vi "funçãoAvaliaçãoAtacante.vi"(9 "balls":T9[](array[typedef]), 10 "Robot in":T4, 11 "IA State":T3={"our_robots"=[], "enemy_robots"=[], "balls"=[], "geometry"={"field_length"=0, "field_width"=0, "goal_width"=0, "goal_depth"=0, "center_circle_radius"=0, "defense_width"=0, "defense_depth"=0, "free_kick_from_defense_dist"=0, "penalty_spot_from_field_line_dist"=0, "penalty_line_from_spot_dist"=0, "half_moon_depth"=0, "half_moon_width"=0}, "IA Judge"={"stage"="", "command"="", "our_goalie_id"=0.0, "enemy_goalie_id"=0.0, "command enum"=enum."Halt", "Time"=enum."Azul"}, "Received Timestamp"=timestamp(0 s since 1904-01-01), "Events"={"Touch"=FALSE, "id touch"=0.0, "Ball out of \nVision"=FALSE, "Ball inside \nGoalie area"=FALSE, "Robot not responding"=FALSE, "Robots responding status"=[1.0, 1.0, 1.0, 1.0, 1.0, 1.0], "Enemy Ball \nPossession"=FALSE, "Id ini Possession"=0.0, "Ball Possesion"=FALSE, "Id Possesion"=0.0, "Ball at\nour goal side"=FALSE, "Ball at\ntouchline"=FALSE, "Ball at\nenemy goal side"=FALSE}}) -> (2 "Parede":T1(ring), 3 "Estado_Atacante":T2(ring))   [LabVIEW 2018]
doc: "Função que avalia o estado do atacante,"
uses:
  Intel/Functions Enum.ctl
  Intel/AttackerStates.ctl
  Path Planning/RRT/PathDest.ctl
  Path Planning/RRT/PathDests.ctl
  Core/AI Robot.ctl
  Core/AI Ball.ctl
  Core/Field Size.ctl
  Intel/Command Enum.ctl
  Core/AI Judge.ctl
  Util/Events/Events.ctl
  Core/AI Input.ctl
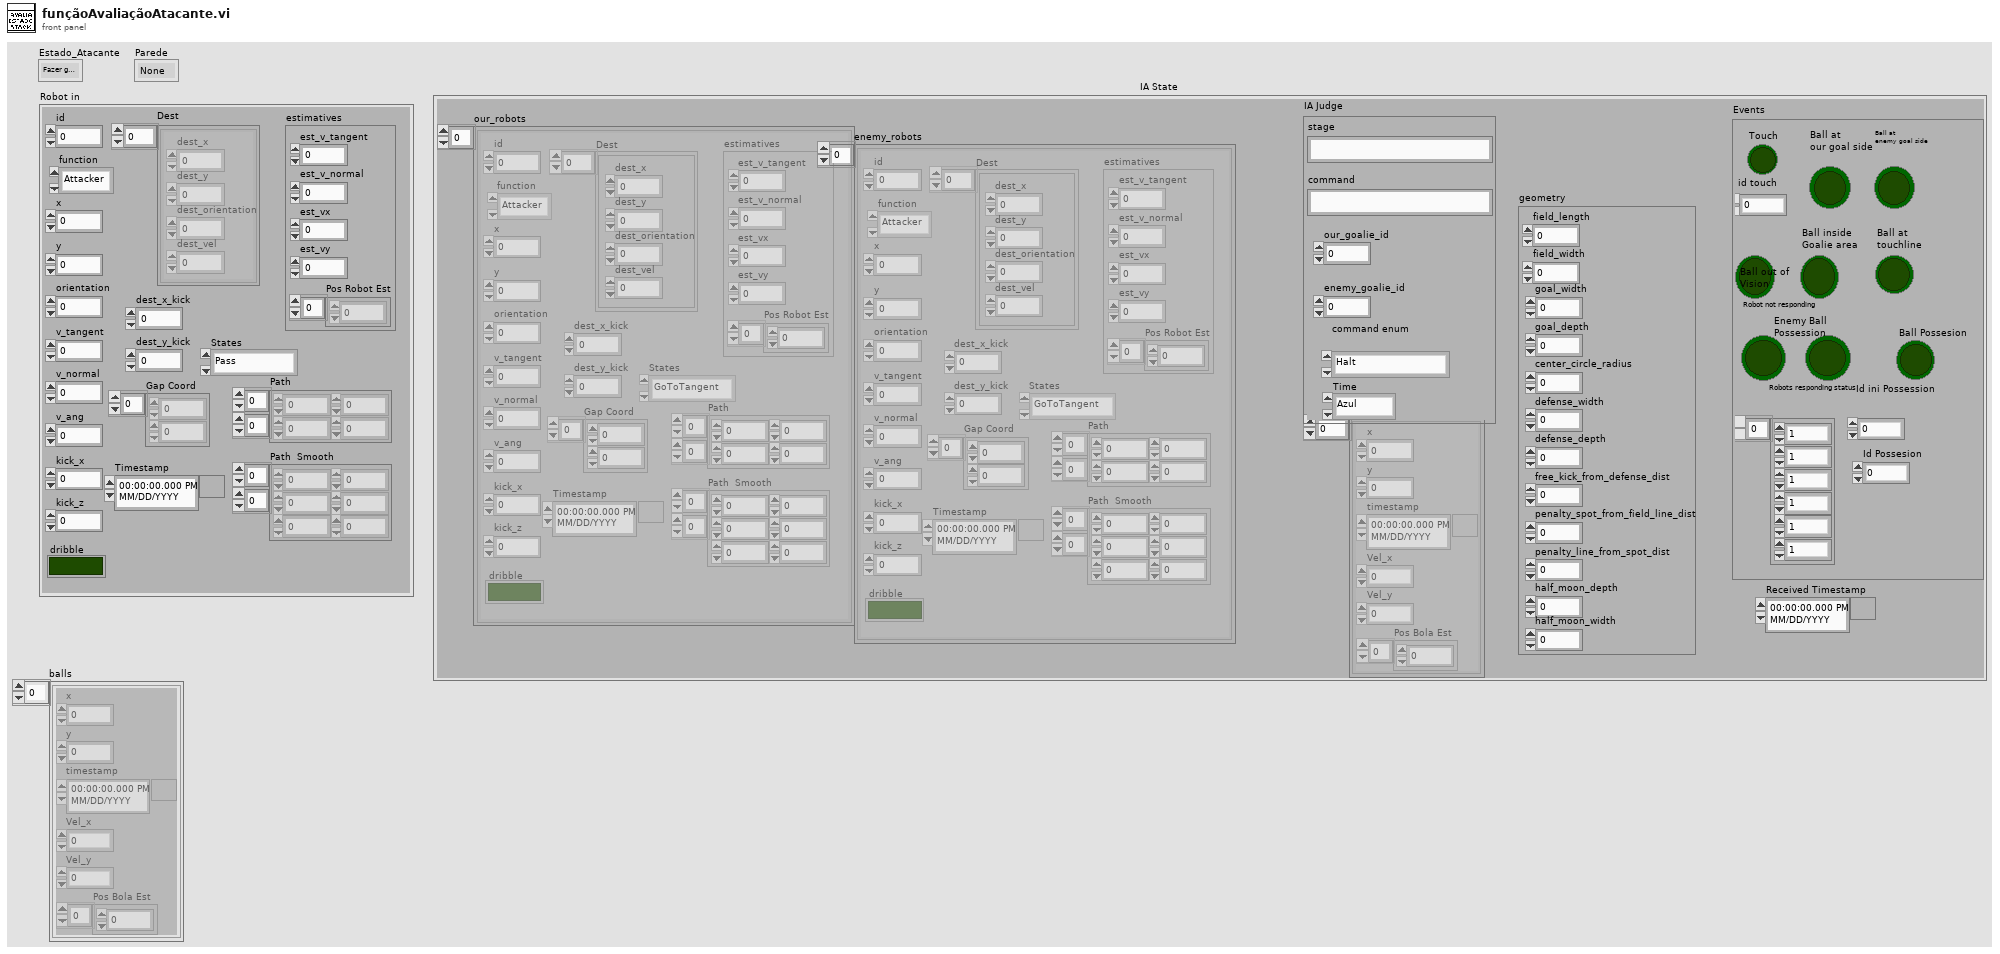
[diagram p1: front panel]
types:
  T1 = enum16{"None", "Frente", "Trás", "Cima", "Baixo"}
  T2 = enum16{"Fazer gol pela lateral", "Tirar bola da parede", "Default", "Sair da parede", "Spin igual a um louco"}
  T3 = typedef "AI Input.ctl" = cluster{"our_robots":T4[], "enemy_robots":T4[], "balls":T9[], "geometry":T10, "IA Judge":T11, "Received Timestamp":timestamp, "Events":T13}
  T4 = typedef "AI Robot.ctl" = cluster{"id":u32, "function":T5, "x":dbl, "y":dbl, "orientation":dbl, "v_tangent":dbl, "v_normal":dbl, "v_ang":dbl, "kick_x":dbl, "kick_z":dbl, "dribble":bool, "Timestamp":timestamp, "estimatives":cluster{"est_v_tangent":dbl, "est_v_normal":dbl, "est_vx":dbl, "est_vy":dbl, "Pos Robot Est":dbl[]}, "dest_x_kick":dbl, "dest_y_kick":dbl, "Gap Coord":dbl[], "States":T6, "Path ":dbl[][], "Path  Smooth":dbl[][], "Dest":T7}
  T5 = typedef "Functions Enum.ctl" = enum16{"Attacker", "Goalie", "Defender", "Striker", "Goto 0", "Dummy", "Kicker", "ZigZag"}
  T6 = typedef "AttackerStates.ctl" = enum16{"Pass", "GoToTangent", "BallGetting", "GoToKick", "Rotate anti-clockwise", "Rotate Clockwise", ""}
  T7 = typedef "PathDests.ctl" = T8[]
  T8 = typedef "PathDest.ctl" = cluster{"dest_x":dbl, "dest_y":dbl, "dest_orientation":dbl, "dest_vel":dbl}
  T9 = typedef "AI Ball.ctl" = cluster{"x":dbl, "y":dbl, "timestamp":timestamp, "Vel_x":dbl, "Vel_y":dbl, "Pos Bola Est":dbl[]}
  T10 = typedef "Field Size.ctl" = cluster{"field_length":u32, "field_width":u32, "goal_width":u32, "goal_depth":u32, "center_circle_radius":u32, "defense_width":u32, "defense_depth":u32, "free_kick_from_defense_dist":u32, "penalty_spot_from_field_line_dist":u32, "penalty_line_from_spot_dist":u32, "half_moon_depth":u32, "half_moon_width":u32}
  T11 = typedef "AI Judge.ctl" = cluster{"stage":string, "command":string, "our_goalie_id":dbl, "enemy_goalie_id":dbl, "command enum":T12, "Time":enum16{"Azul", "Amarelo"}}
  T12 = typedef "Command Enum.ctl" = enum16{"Halt", "Stop", "Force Start", "PKA Normal Start", "Prepare Kickoff Ally", "PKE Normal Start", "Prepare Kickoff Enemy", "Prepare Penalty Ally", "PPA Normal Start", "Prepare Penalty Enemy", "PPE Normal Start", "Ball Placement Enemy Up", "Ball Placement Enemy Down", "Ball Placement Ally Up", "Ball Placement Ally Mid", "Ball Placement Ally Down", "Indirect Free Enemy", "Indirect Free Ally", "Timeout Enemy", "Timeout Ally", "Goal Enemy", "Goal Ally", "Normal Half Time", "Extra Time Break", "Extra Half Time", "None", "Post Game"}
  T13 = typedef "Events.ctl" = cluster{"Touch":bool, "id touch":dbl, "Ball out of \nVision":bool, "Ball inside \nGoalie area":bool, "Robot not responding":bool, "Robots responding status":dbl[], "Enemy Ball \nPossession":bool, "Id ini Possession":dbl, "Ball Possesion":bool, "Id Possesion":dbl, "Ball at\nour goal side":bool, "Ball at\ntouchline":bool, "Ball at\nenemy goal side":bool}
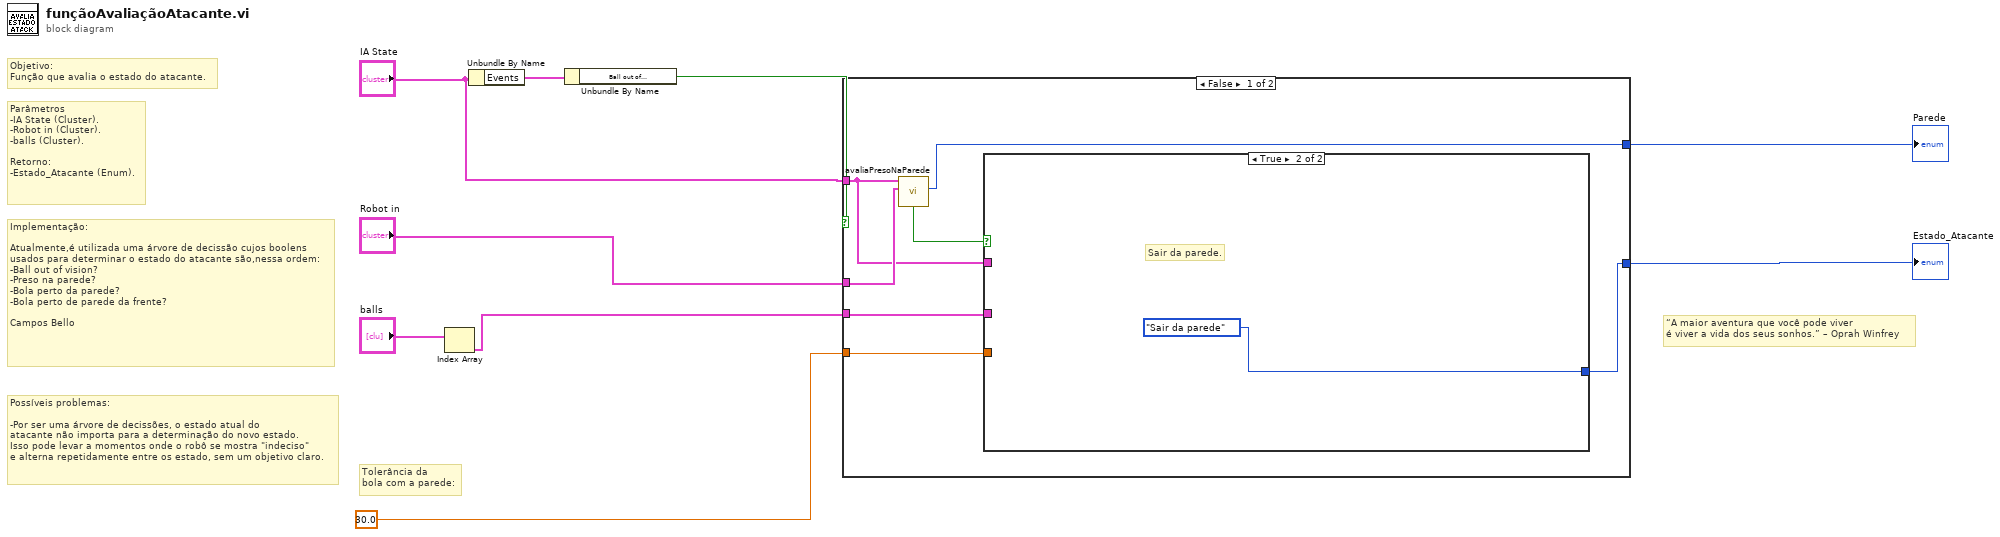
[diagram p0: block diagram]
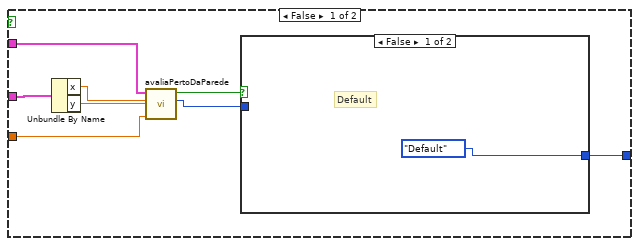
[diagram p2: hidden frame]
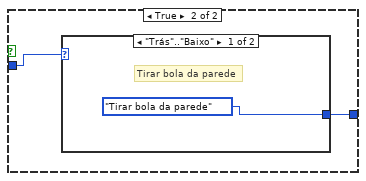
[diagram p3: hidden frame]
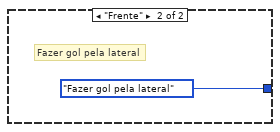
[diagram p4: hidden frame]
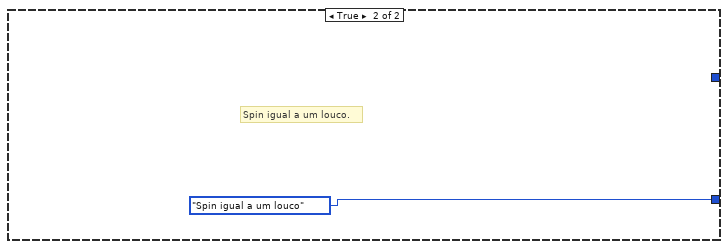
[diagram p5: hidden frame]
diagram:
  # "“A maior aventura que você pode viver\né viver a vida dos seus sonhos.” – Oprah Winfrey"
  # "Possíveis problemas:\n\n-Por ser uma árvore de decissões, o estado atual do\natacante não importa para a determinação do novo estado. \nIsso pode levar a momentos onde o robô se mostra \"indeciso\"\ne alterna repetidamente entre os estado, sem um objetivo claro."
  # "Implementação:\n\nAtualmente,é utilizada uma árvore de decissão cujos boolens\nusados para determinar o estado do atacante são,nessa ordem:\n-Ball out of vision?\n-Preso na parede?\n-Bola perto da parede?\n-Bola perto de parede da frente?\n\nCampos Bello"
  # "Parâmetros\n-IA State (Cluster).\n-Robot in (Cluster).\n-balls (Cluster).\n\nRetorno:\n-Estado_Atacante (Enum)."
  # "Objetivo:\nFunção que avalia o estado do atacante."
  # "Tolerância da\nbola com a parede:"
  n1 = Index Array(array="balls") -> (element=w5:T9)  [unwired: 1 in]
  n2 = Unbundle By Name("IA State") -> ("Events"=w9:T13)
  n3 = Unbundle By Name(w9) -> ("Ball out of \nVision"=w8:bool)
  n4 = case shown="False" w8 {
    tunnel: "IA State" -> [w13 _]
    tunnel: w5 -> [w15 _]
    tunnel: "Robot in" -> [w14 _]
    tunnel: 30.0 -> [w12 _]
    tunnel: [w11 T2."Spin igual a um louco" ("Enum")] -> w2
    tunnel: [w10 _] -> w1
    frame False {
      n5 = call "avaliaPresoNaParede.vi"("Robot in"=w14, "IA State"=w13) -> ("Parede"=w10:T1, "Preso na parede?"=w16:bool)  [unwired: 8 in]
      n6 = case shown="True" w16 {
        tunnel: w15 -> [w24 _]
        tunnel: w13 -> [w21 _]
        tunnel: w12 -> [w20 _]
        tunnel: [w17 T2."Sair da parede" ("Enum")] -> w11
        frame False {
          n7 = Unbundle By Name(w24) -> ("x"=w23:dbl, "y"=w22:dbl)
          n8 = call "avaliaPertoDaParede.vi"("Distância"=w20, "Y"=w22, "X"=w23, "IA State"=w21) -> ("Enum"=w18:T1, "Perto de parede?"=w19:bool)  [unwired: 6 in]
          n9 = case shown="False" w19 {
            tunnel: w18 -> [_ w27]
            tunnel: [T2."Default" ("Enum") w26] -> w17
            frame False {
              # "Default"
            }
            frame True {
              n10 = case shown="\"Trás\"..\"Baixo\"" w27 {
                tunnel: [T2."Tirar bola da parede" ("Enum") T2."Fazer gol pela lateral" ("Enum")] -> w26
                frame "Trás".."Baixo" {
                  # "Tirar bola da parede"
                }
                frame "Frente" {
                  # "Fazer gol pela lateral"
                }
              }
            }
          }
        }
        frame True {
          # "Sair da parede."
        }
      }
    }
    frame True {
      # "Spin igual a um louco."
    }
  }
  "Estado_Atacante" <- w2
  "Parede" <- w1
